vi "initializeValveDigital-v02.vi"(11 "daq_do":tag="Dev1/ai0:1") -> (2 "ValveSetTo":u16)   [LabVIEW 2015]
uses:
  <vilib>/DAQmx/write.llb/DAQmx Write (Digital 1D Bool NChan 1Samp 1Line).vi
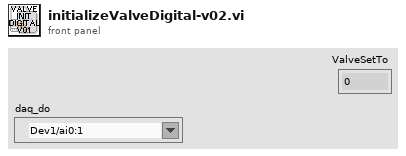
[diagram p1: front panel]
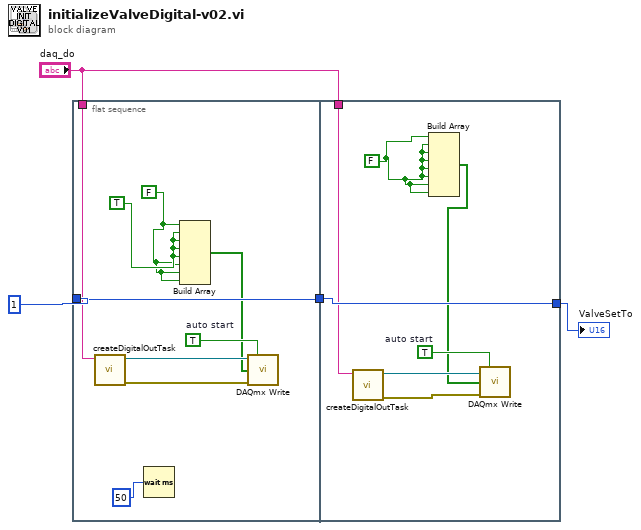
[diagram p0: block diagram]
diagram:
  n1 = flat-sequence {
    tunnel: "daq_do" -> [w9]
    tunnel: u16 1 -> [w8]
    tunnel: [w8] -> w4
    tunnel: w4 -> [w20]
    tunnel: [w20] -> w3
    tunnel: "daq_do" -> [w16]
    frame #0 {
      w5 = FALSE
      w6 = TRUE
      w12 = TRUE  # auto start
      n2 = call "createDigitalOutTask.vi"("daq_do"=w9) -> ("error out"=w10:errorcluster, "task out"=w11:refnum<k21>)  [unwired: 9 in]
      n3 = Wait (ms)(milliseconds to wait=u32 50) -> ()  [unwired: 1 out]
      n4 = Build Array(w5, w6, w6, w6, w6, w5, w5, w5) -> (w7:bool[])
      n5 = call-poly <vilib>:"DAQmx Write.vi"("task/channels in"=w11, "auto start"=w12, "data"=w7, "error in"=w10) -> ()  [unwired: 9 in, 3 out]
    }
    frame #1 {
      w14 = FALSE
      w19 = TRUE  # auto start
      n6 = call "createDigitalOutTask.vi"("daq_do"=w16) -> ("error out"=w17:errorcluster, "task out"=w18:refnum<k21>)  [unwired: 9 in]
      n7 = Build Array(w14, w14, w14, w14, w14, w14, w14, w14) -> (w15:bool[])
      n8 = call-poly <vilib>:"DAQmx Write.vi"("task/channels in"=w18, "auto start"=w19, "data"=w15, "error in"=w17) -> ()  [unwired: 9 in, 3 out]
    }
  }
  "ValveSetTo" <- w3
